vi "peakFinding getAnnotationData.vi"(5 "Color Box":u32(colorbox)=16711680, 7 "name":string="peak", 9 "getIdxArray":i32[](array[numeric]), 10 "yData":dbl[](array[numeric]), 11 "xData":dbl[](array[numeric])) -> (3 "AnntData":T1(array[cluster]))   [LabVIEW 2018]
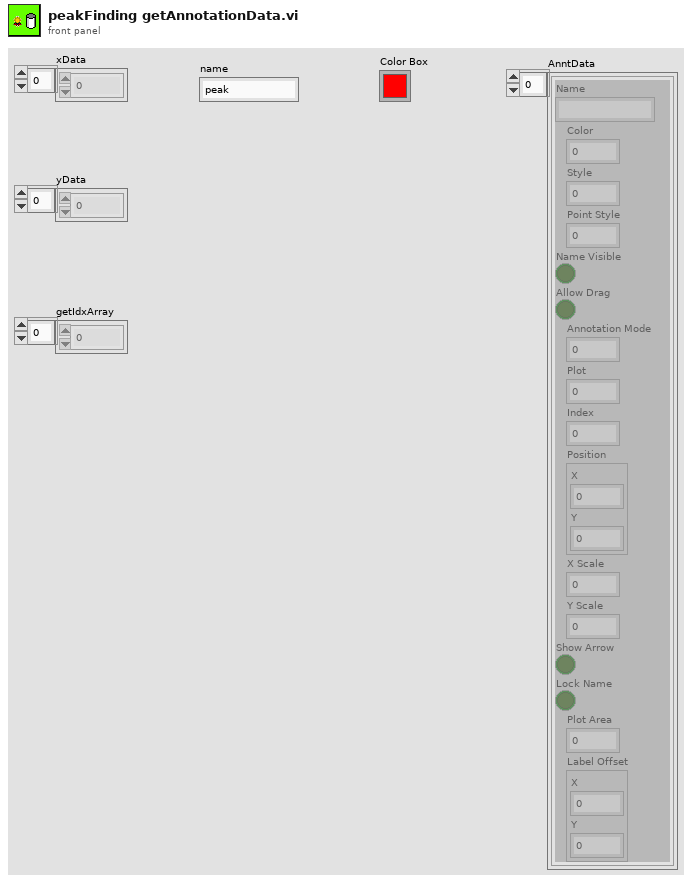
[diagram p1: front panel]
types:
  T1 = cluster{"Name":string, "Color":i32, "Style":u8, "Point Style":i32, "Name Visible":bool, "Allow Drag":bool, "Annotation Mode":u32, "Plot":i32, "Index":i32, "Position":cluster{"X":dbl, "Y":dbl}, "X Scale":u32, "Y Scale":u32, "Show Arrow":bool, "Lock Name":bool, "Plot Area":i32, "Label Offset":cluster{"X":dbl, "Y":dbl}}[]
  T2 = cluster{"Name":string, "Color":i32, "Style":u8, "Point Style":i32, "Name Visible":bool, "Allow Drag":bool, "Annotation Mode":u32, "Plot":i32, "Index":i32, "Position":cluster{"X":dbl, "Y":dbl}, "X Scale":u32, "Y Scale":u32, "Show Arrow":bool, "Lock Name":bool, "Plot Area":i32, "Label Offset":cluster{"X":dbl, "Y":dbl}}
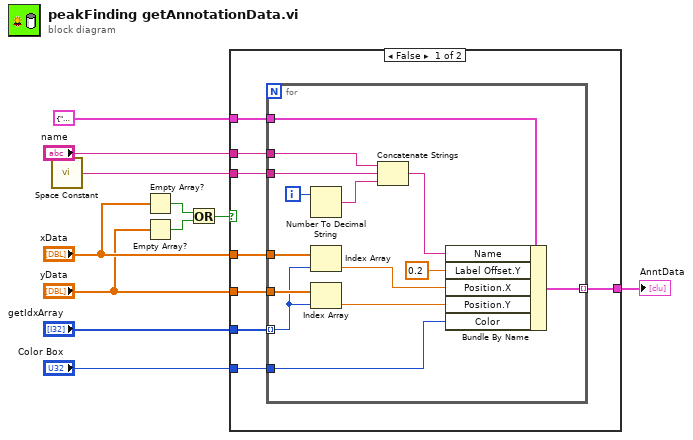
[diagram p0: block diagram]
diagram:
  n1 = call <vilib>:"Space Constant.vi"() -> ("String"=w7:string)
  n2 = Empty Array?(array="xData") -> (empty?=w3:bool)
  n3 = Empty Array?(array="yData") -> (empty?=w2:bool)
  n4 = Or(x=w3, y=w2) -> (x .or. y?=w1:bool)
  n5 = case shown="False" w1 {
    tunnel: T2 {"Name"="", "Color"=16711680, "Style"=0, "Point Style"=2, "Name Visible"=TRUE, "Allow Drag"=FALSE, "Annotation Mode"=0, "Plot"=0, "Index"=0, "Position"={"X"=0.0, "Y"=0.0}, "X Scale"=0, "Y Scale"=0, "Show Arrow"=FALSE, "Lock Name"=TRUE, "Plot Area"=0, "Label Offset"={"X"=0.0, "Y"=0.0}} -> [w19 _]
    tunnel: "getIdxArray" -> [w18 _]
    tunnel: "Color Box" -> [w17 _]
    tunnel: "name" -> [w16 _]
    tunnel: w7 -> [w15 _]
    tunnel: [w14 _] -> w6
    tunnel: "xData" -> [w13 _]
    tunnel: "yData" -> [w12 _]
    frame False {
      n6 = for {
        tunnel: [w31] -> w14 mode=indexing
        tunnel: w18 -> [w29] mode=indexing
        tunnel: w12 -> [w30]
        tunnel: w13 -> [w28]
        tunnel: w19 -> [w27]
        tunnel: w17 -> [w26]
        tunnel: w16 -> [w24]
        tunnel: w15 -> [w25]
        i -> [w32]
        n7 = Number To Decimal String(number=w32) -> (decimal integer string=w23:string)  [unwired: 1 in]
        n8 = Index Array(array=w28, index=w29) -> (element=w21:dbl)
        n9 = Index Array(array=w30, index=w29) -> (element=w20:dbl)
        n10 = Concatenate Strings(w24, w25, w23) -> (w22:string)
        n11 = Bundle By Name(cluster=w27, "Name"=w22, "Label Offset.Y"=0.2, "Position.X"=w21, "Position.Y"=w20, "Color"=w26) -> (w31:T2)
      }
    }
    frame True {
    }
  }
  "AnntData" <- w6
